vi "GetTraverse.vi"(8 "error in (no error)":errorcluster, 11 "VariantTree in":refnum<class "VariantTree__VP.lvclass">) -> (0 "error out":errorcluster, 2 "Traverse":bool, 3 "VariantTree out":refnum<class "VariantTree__VP.lvclass">)   [LabVIEW 2013, in "VariantTree__VP.lvclass"]
uses:
  VariantTree__VP.lvclass
  VariantTree__VP.lvclass/VariantTree__VP.ctl
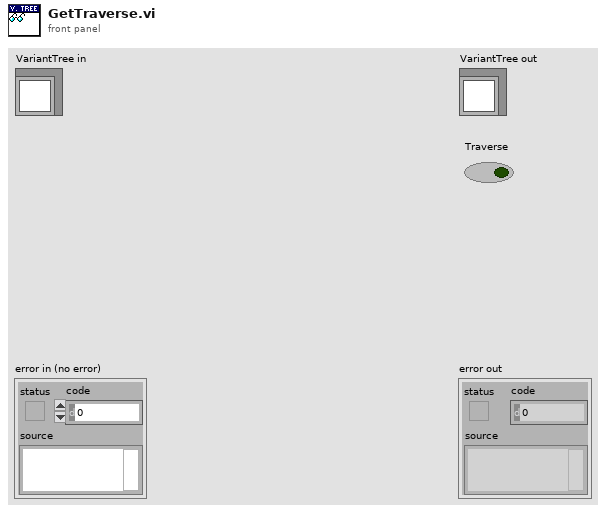
[diagram p1: front panel]
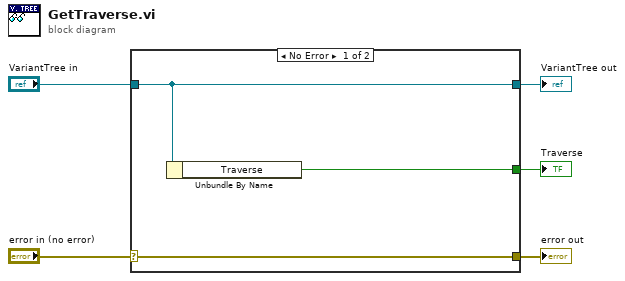
[diagram p0: block diagram]
diagram:
  n1 = case shown="No Error" "error in (no error)" {
    selector: "error in (no error)" -> [w8 w9]
    tunnel: [w8 w9] -> w4
    tunnel: [w7 w10] -> w2
    tunnel: "VariantTree in" -> [w7 w10]
    tunnel: [w6 _] -> w1
    frame No Error {
      n2 = Unbundle By Name(w7) -> ("Traverse"=w6:bool)
    }
    frame Error {
    }
  }
  "error out" <- w4
  "VariantTree out" <- w2
  "Traverse" <- w1
